vi "Get BD Reference.vi"(8 "error in":errorcluster, 11 "VI in":refnum<vi>) -> (0 "error out":errorcluster, 2 "Block Diagram":refnum<vi>, 3 "VI out":refnum<vi>)   [LabVIEW 2019, in "gRPC Template Creation Utility.lvlib"]
uses:
  gRPC Template Creation Utility.lvlib
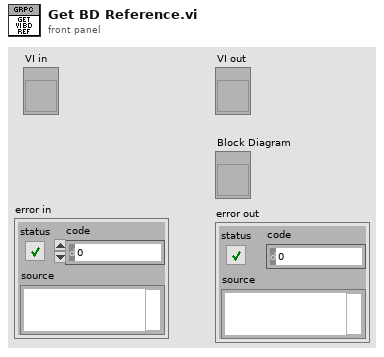
[diagram p1: front panel]
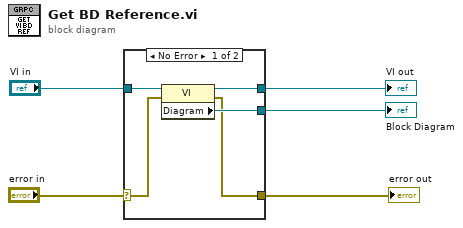
[diagram p0: block diagram]
diagram:
  n1 = case shown="No Error" "error in" {
    selector: "error in" -> [w8 w12]
    tunnel: "VI in" -> [w10 w11]
    tunnel: [w9 w11] -> w2
    tunnel: [w7 _] -> w3
    tunnel: [w6 w12] -> w1
    frame No Error {
      n2 = property class="VI"(reference=w10, error in=w8) -> (reference out=w9:refnum<vi>, error out=w6:errorcluster, "Diagram"=w7:refnum<vi>)
    }
    frame Error {
    }
  }
  "Block Diagram" <- w3
  "VI out" <- w2
  "error out" <- w1
